vi "Read Channel URL list.vi"(8 "error in (no error)":errorcluster, 11 "TDMS datalogger editor node in":refnum<class "TDMS datalogger editor node.lvclass">) -> (0 "error out":errorcluster, 2 "URLs":string[](array[string]), 3 "TDMS datalogger editor node out":refnum<class "TDMS datalogger editor node.lvclass">)   [LabVIEW 2013, in "TDMS datalogger editor node.lvclass"]
uses:
  TDMS datalogger editor node.lvclass
  <vilib>/NI/Tag Bus Data Framework/Configuration Editor/Classes/Module editor node/module editor node.lvclass
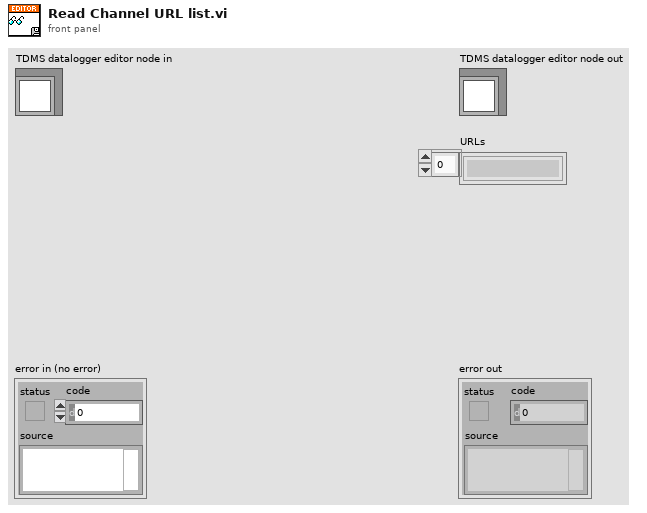
[diagram p1: front panel]
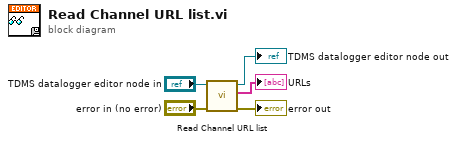
[diagram p0: block diagram]
diagram:
  n1 = call-parent "Read Channel URL list.vi"("error in"="error in (no error)", "Module Editor Node in"="TDMS datalogger editor node in") -> ("error out"=→"error out":errorcluster, "URLs"=→"URLs":string[], "Module Editor Node out"=→"TDMS datalogger editor node out":refnum<class "TDMS datalogger editor node.lvclass">)  [unwired: 7 in]
